vi "PID for Pressure.vi"(0 "ControlArray":T1(array[cluster])=[{"Name"="Volt_Direct", "PI Far->Close"=[], "FFinfo"={"FF_m"=0.0, "FF_b"=0.0}, "Limits"={"StepSize"=1e-05, "Max"=10.0, "Min"=0.0, "IndMin"=0.0}}, {"Name"="Volt_Flow", "PI Far->Close"=[], "FFinfo"={"FF_m"=0.0, "FF_b"=0.0}, "Limits"={"StepSize"=1e-05, "Max"=10.0, "Min"=0.0, "IndMin"=0.0}}, {"Name"="Volt_Speed", "PI Far->Close"=[], "FFinfo"={"FF_m"=0.0, "FF_b"=0.0}, "Limits"={"StepSize"=1e-05, "Max"=10.0, "Min"=0.0, "IndMin"=0.0}}, {"Name"="Pres_Direct", "PI Far->Close"=[], "FFinfo"={"FF_m"=0.0, "FF_b"=0.0}, "Limits"={"StepSize"=1e-05, "Max"=10.0, "Min"=0.0, "IndMin"=0.0}}, {"Name"="Pres_Flow", "PI Far->Close"=[], "FFinfo"={"FF_m"=0.0, "FF_b"=0.0}, "Limits"={"StepSize"=1e-05, "Max"=10.0, "Min"=0.0, "IndMin"=0.0}}, {"Name"="Pres_Speed", "PI Far->Close"=[], "FFinfo"={"FF_m"=0.0, "FF_b"=0.0}, "Limits"={"StepSize"=1e-05, "Max"=10.0, "Min"=0.0, "IndMin"=0.0}}, {"Name"="CMD_Direct", "PI Far->Close"=[], "FFinfo"={"FF_m"=0.0, "FF_b"=0.0}, "Limits"={"StepSize"=1e-05, "Max"=10.0, "Min"=0.0, "IndMin"=0.0}}, {"Name"="CMD_Flow", "PI Far->Close"=[], "FFinfo"={"FF_m"=0.0, "FF_b"=0.0}, "Limits"={"StepSize"=1e-05, "Max"=10.0, "Min"=0.0, "IndMin"=0.0}}, {"Name"="CMD_Speed", "PI Far->Close"=[], "FFinfo"={"FF_m"=0.0, "FF_b"=0.0}, "Limits"={"StepSize"=1e-05, "Max"=10.0, "Min"=0.0, "IndMin"=0.0}}], 1 "NeedleValve":bool, 3 "Feedback":dbl[](array[numeric]), 5 "CommandCluster":T2, 9 "VandPLimits":dbl[](array[numeric]), 11 "Run?":bool, 13 "Controller?":bool) -> (4 "PIdata":dbl[](array[numeric]), 8 "Output":dbl)   [LabVIEW 2013]
uses:
  TypeDef/Command Cluster.ctl
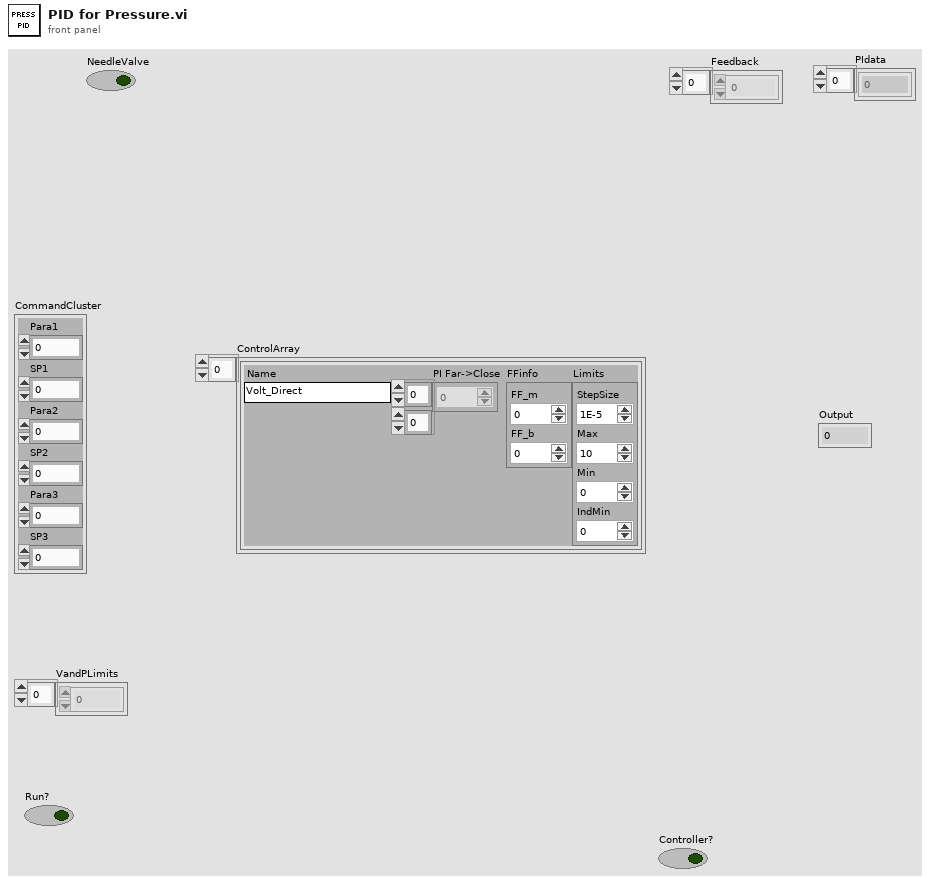
[diagram p1: front panel]
types:
  T1 = cluster{"Name":string, "PI Far->Close":dbl[][], "FFinfo":cluster{"FF_m":dbl, "FF_b":dbl}, "Limits":cluster{"StepSize":dbl, "Max":dbl, "Min":dbl, "IndMin":dbl}}[]
  T2 = typedef "Command Cluster.ctl" = cluster{"Para1":i32, "SP1":dbl, "Para2":i32, "SP2":dbl, "Para3":i32, "SP3":dbl}
  T3 = cluster{"Name":string, "PI Far->Close":dbl[][], "FFinfo":cluster{"FF_m":dbl, "FF_b":dbl}, "Limits":cluster{"StepSize":dbl, "Max":dbl, "Min":dbl, "IndMin":dbl}}
  T4 = cluster{"StepSize":dbl, "Max":dbl, "Min":dbl, "IndMin":dbl}
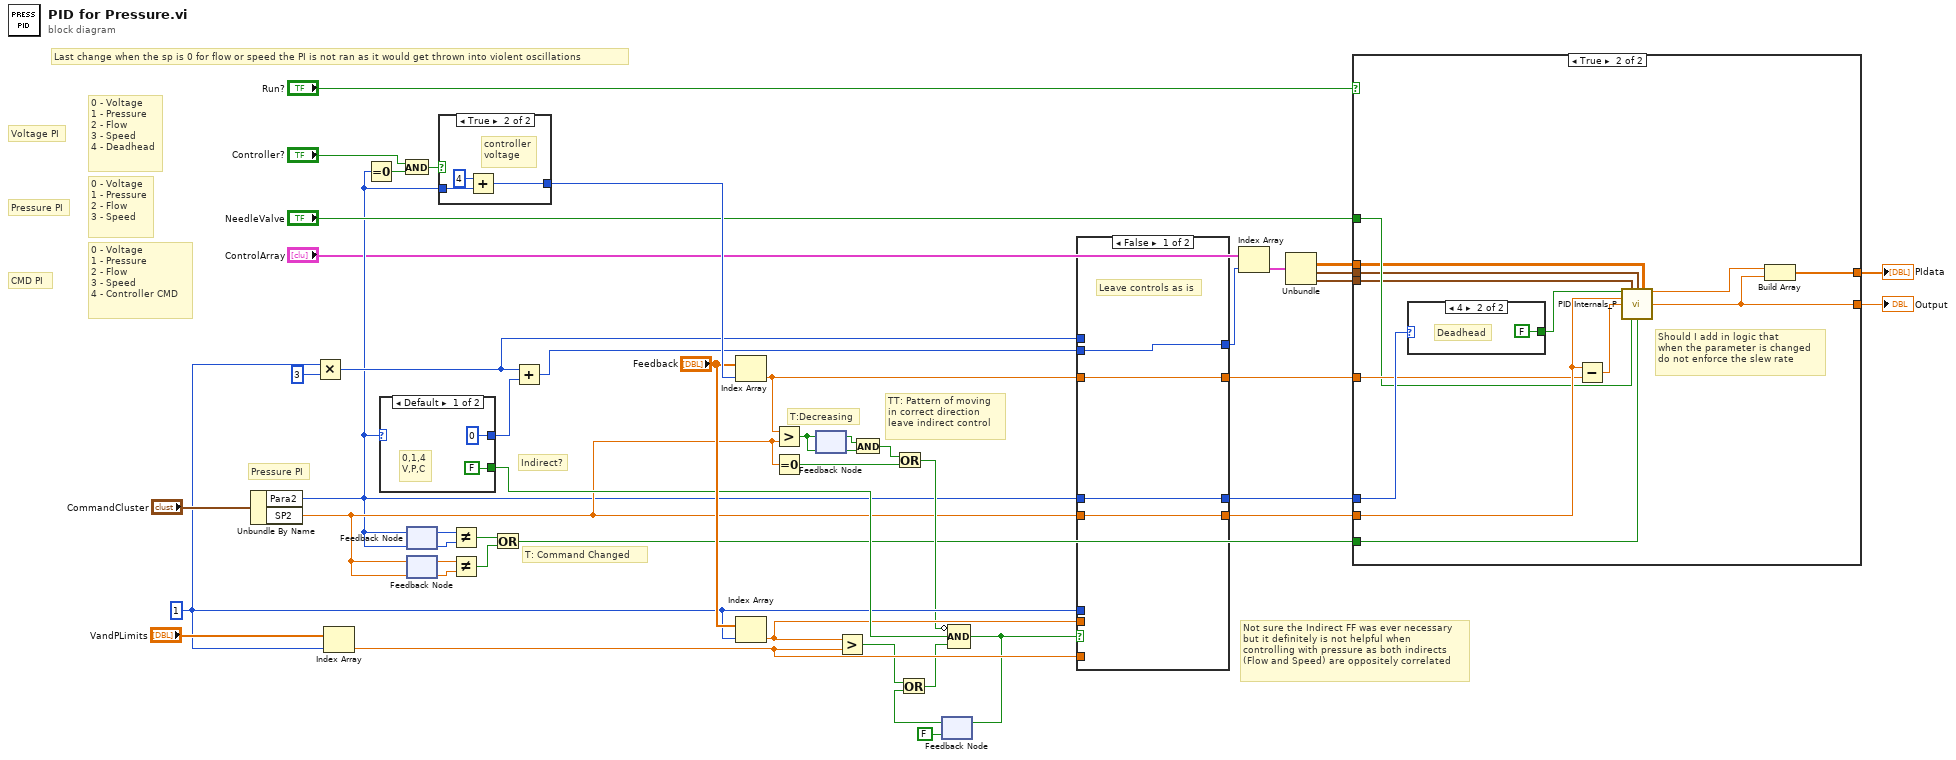
[diagram p0: block diagram]
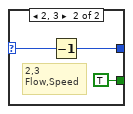
[diagram p4: hidden frame]
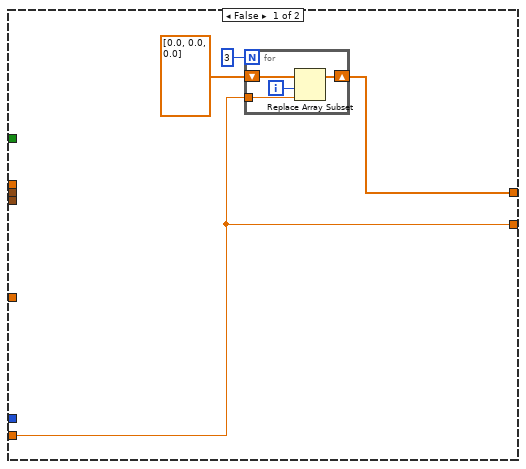
[diagram p5: hidden frame]
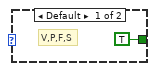
[diagram p6: hidden frame]
diagram:
  w31 = 1 ("CtrlIndex")
  # "T: Command Changed"
  # "Pressure PI"
  # "Not sure the Indirect FF was ever necessary\nbut it definitely is not helpful when\ncontrolling with pressure as both indirects\n(Flow and Speed) are oppositely correlated"
  # "TT: Pattern of moving\nin correct direction\nleave indirect control"
  # "T:Decreasing"
  # "Indirect?"
  # "Last change when the sp is 0 for flow or speed the PI is not ran as it would get thrown into violent oscillations"
  # "CMD PI"
  # "Pressure PI"
  # "Voltage PI"
  # "0 - Voltage\n1 - Pressure\n2 - Flow\n3 - Speed\n4 - Controller CMD"
  # "0 - Voltage\n1 - Pressure\n2 - Flow\n3 - Speed"
  # "0 - Voltage\n1 - Pressure\n2 - Flow\n3 - Speed\n4 - Deadhead"
  n1 = Unbundle By Name("CommandCluster") -> ("Para2"=w11:i32, "SP2"=w13:dbl)
  n2 = Multiply(x=w31, y=3) -> (x*y=w26:i32)
  n3 = Index Array(array="VandPLimits", index=w31) -> (element=w30:dbl)
  n4 = Equal To 0?(x=w11) -> (x = 0?=w39:bool)
  n5 = case shown="Default" w11 {
    selector: w11 -> [_ w51]
    tunnel: [0 w50] -> w41
    tunnel: [FALSE TRUE] -> w32
    frame Default {
      # "0,1,4\nV,P,C"
    }
    frame 2, 3 {
      # "2,3\nFlow,Speed"
      n6 = Decrement(x=w51) -> (x-1=w50:i32)
    }
  }
  n7 = And(x="Controller?", y=w39) -> (x .and. y?=w40:bool)
  n8 = feedback-in #1(w11) -> ()
  n9 = feedback #1(w11) -> (w10:i32)
  n10 = feedback #2(w13) -> (w12:dbl)
  n11 = feedback-in #2(w13) -> ()
  n12 = case shown="True" w40 {
    tunnel: w11 -> [w52 w55]
    tunnel: [w52 w53] -> w36
    frame False {
      # "pump\nvoltage"
    }
    frame True {
      # "controller\nvoltage"
      n13 = Add(x=4, y=w55) -> (x+y=w53:i32)
    }
  }
  n14 = Not Equal?(x=w10, y=w11) -> (x != y?=w9:bool)
  n15 = Not Equal?(x=w12, y=w13) -> (x != y?=w8:bool)
  n16 = Or(x=w9, y=w8) -> (x .or. y?=w7:bool)
  n17 = Add(x=w26, y=w41) -> (x+y=w25:i32)
  n18 = Index Array(array="Feedback", index=w36) -> (element=w28:dbl)
  n19 = Index Array(array="Feedback", index=w31) -> (element=w29:dbl)
  n20 = Greater?(x=w28, y=w13) -> (0:w34:bool)
  n21 = Equal To 0?(x=w13) -> (x = 0?=w24:bool)
  n22 = feedback #3(w34) -> (w33:bool)
  n23 = feedback-in #3(w34) -> ()
  n24 = Greater?(x=w29, y=w30) -> (0:w19:bool)
  n25 = And(x=w33, y=w34) -> (x .and. y?=w23:bool)
  n26 = Or(x=w23, y=w24) -> (x .or. y?=w22:bool)
  n27 = feedback #4(FALSE) -> (w20:bool)
  n28 = Or(x=w19, y=w20) -> (x .or. y?=w17:bool)
  n29 = Compound Arithmetic op=AND(invert w22, w32, w17) -> (w18:bool)
  n30 = feedback-in #4(w18) -> ()
  n31 = case shown="False" w18 {
    tunnel: w11 -> [w59 _]
    tunnel: w13 -> [w58 _]
    tunnel: [w59 w62] -> w14
    tunnel: [w58 w63] -> w16
    tunnel: w28 -> [w57 _]
    tunnel: [w57 w61] -> w27
    tunnel: w25 -> [w56 _]
    tunnel: [w56 w60] -> w5
    tunnel: w29 -> [_ w61]
    tunnel: w30 -> [_ w63]
    tunnel: w31 -> [_ w62]
    tunnel: w26 -> [_ w60]
    frame False {
      # "Leave controls as is"
    }
    frame True {
      # "Change from indirect\nto direct control due\nto over limit"
    }
  }
  n32 = Index Array(array="ControlArray", index=w5) -> (element=w4:T3)
  n33 = Unbundle(w4) -> ("PI Far->Close"=w3:dbl[][], "FFinfo"=w1:cluster{"FF_m":dbl, "FF_b":dbl}, "Limits"=w2:T4)  [unwired: 1 out]
  n34 = case shown="True" "Run?" {
    tunnel: w14 -> [_ w81]
    tunnel: w16 -> [w67 w83]
    tunnel: [w67 w80] -> w45
    tunnel: [w65 w84] -> w44
    tunnel: w27 -> [_ w78]
    tunnel: "NeedleValve" -> [_ w77]
    tunnel: w7 -> [_ w75]
    tunnel: w3 -> [_ w72]
    tunnel: w2 -> [_ w74]
    tunnel: w1 -> [_ w73]
    frame False {
      n35 = for {
        N: 3 -> [_]
        shift-right: [w70] -> w65
        shift-left: dbl[] [0.0, 0.0, 0.0] -> [w71]
        tunnel: w67 -> [w68]
        i -> [w69]
        n36 = Replace Array Subset(array=w71, new element=w68, index=w69) -> (w70:dbl[])
      }
    }
    frame True {
      # "Should I add in logic that\nwhen the parameter is changed\ndo not enforce the slew rate"
      n37 = case shown="4" w81 {
        tunnel: [TRUE FALSE] -> w76
        frame Default {
          # "V,P,F,S"
        }
        frame 4 {
          # "Deadhead"
        }
      }
      n38 = Subtract(x=w83, y=w78) -> (x-y=w82:dbl)
      n39 = call "PID Internals_P.vi"("Run PI?"=w76, "LimitCluster"=w74, "FFcluster"=w73, "PI Far->Close2"=w72, "SP"=w83, "Error"=w82, "NeedleValve"=w77, "CmdChanged"=w75) -> ("SlewIndex"=w79:dbl, "Output"=w80:dbl)  [unwired: 6 in]
      n40 = Build Array(w79, w80) -> (w84:dbl[])
    }
  }
  "Output" <- w45
  "PIdata" <- w44
